vi "ActFollowRelativeTrajectory.vi"(7 "Orientation":T1, 9 "End Rotation":dbl, 10 "Trajectory":T2 {"States"."POSE"."ROTATION"."SIN" format="%13.4f"; "States"."POSE"."ROTATION"."COS" format="%13.4f"; "States"."POSE"."ROTATION"."VALUE" format="%13.4f"; "States"."POSE"."TRANSLATION"."Y" format="%14.3f"; "States"."POSE"."TRANSLATION"."X" format="%14.3f"; "TotalTImeSecs" format="%20.3f"}, 11 "FirstTime":bool) -> (0 "Done":bool, 1 "ASpeedDemand":dbl, 2 "YSpeedDemand":dbl, 3 "XSpeedDemand":dbl)   [LabVIEW 2020]
uses:
  <vilib>/Rock Robotics/WPI/ThirdParty/JAS_Junk/TrajLib/TypeDef/TRAJECTORY.ctl
  <vilib>/Rock Robotics/WPI/ThirdParty/JAS_Junk/TrajLib/TypeDef/TRAJ_STATE.ctl
  <vilib>/Rock Robotics/WPI/ThirdParty/JAS_Junk/TrajLib/TypeDef/POSE2D.ctl
  <vilib>/Rock Robotics/WPI/ThirdParty/JAS_Junk/TrajLib/TypeDef/TRANSLATION2D.ctl
  <vilib>/Rock Robotics/WPI/ThirdParty/JAS_Junk/TrajLib/TypeDef/ROTATION2D.ctl
  <vilib>/Rock Robotics/WPI/ThirdParty/JAS_Junk/TrajLib/Conv_Deg_Radians.vi
  <vilib>/Rock Robotics/WPI/ThirdParty/JAS_Junk/TrajLib/Rotation2d_CreateAngle.vi
  <vilib>/Rock Robotics/WPI/ThirdParty/JAS_Junk/TrajLib/Trajectory_Library.lvlib
  Autonomous/TrajectoryOrientation.ctl
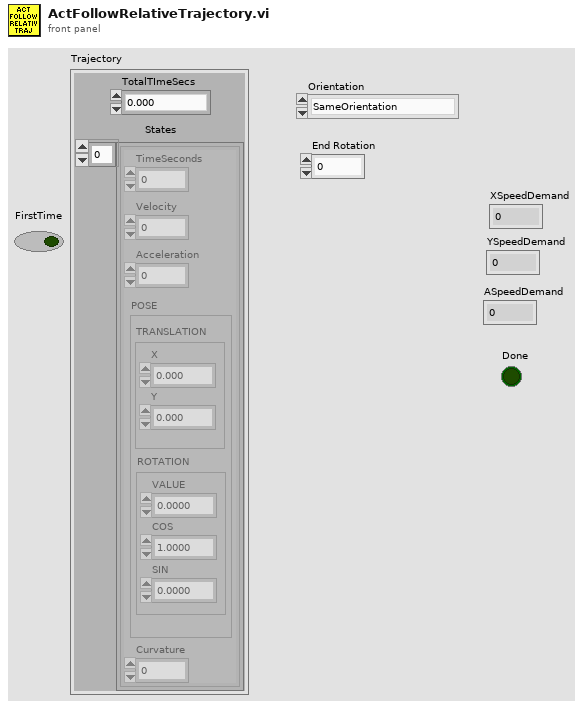
[diagram p1: front panel]
types:
  T1 = typedef "TrajectoryOrientation.ctl" = enum16{"SameOrientation", "RotateToEndOrientation"}
  T2 = typedef "Trajectory_Library.lvlib/TRAJECTORY.ctl" = cluster{"TotalTImeSecs":dbl, "States":T3[]}
  T3 = typedef "Trajectory_Library.lvlib/TRAJ_STATE.ctl" = cluster{"TimeSeconds":dbl, "Velocity":dbl, "Acceleration":dbl, "POSE":T4, "Curvature":dbl}
  T4 = typedef "Trajectory_Library.lvlib/POSE2D.ctl" = cluster{"TRANSLATION":T5, "ROTATION":T6}
  T5 = typedef "Trajectory_Library.lvlib/TRANSLATION2D.ctl" = cluster{"X":dbl, "Y":dbl}
  T6 = typedef "Trajectory_Library.lvlib/ROTATION2D.ctl" = cluster{"VALUE":dbl, "COS":dbl, "SIN":dbl}
  T7 = typedef "Trajectory_Library.lvlib/SWERVE_DRIVE_ODOMETRY.ctl" = cluster{"POSE":T4, "GyroOffset":T6, "PreviousAngle":T6, "PrevModulePositions":T8[], "NumModules":i32}
  T8 = typedef "Trajectory_Library.lvlib/SWERVE_DRIVE_MODULE_POSITION.ctl" = cluster{"Distance":dbl, "Angle":T6, "P":bool}
  T9 = typedef "Trajectory_Library.lvlib/SWERVE_DRIVE_KINEMATICS.ctl" = cluster{"NumModules":i32, "InverseKinematics":T10, "ForwardKinematics":T10, "Modules":T5[], "PrevCoR":T5, "SavedModuleStates":T11[]}
  T10 = typedef "NI_Matrix.lvlib/RealMatrix.ctl" = dbl[][]
  T11 = typedef "Trajectory_Library.lvlib/SWERVE_DRIVE_MODULE_STATE.ctl" = cluster{"Speed":dbl, "Angle":T6}
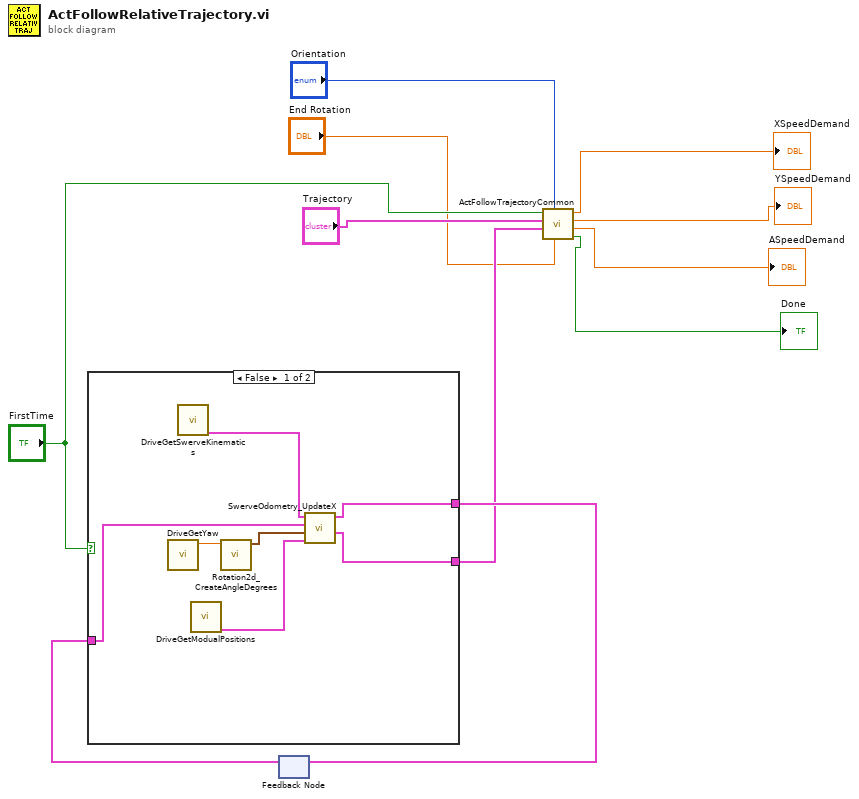
[diagram p0: block diagram]
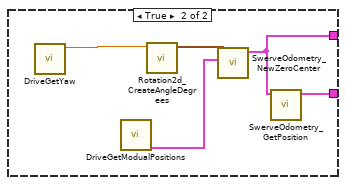
[diagram p2: hidden frame]
diagram:
  n1 = feedback #1() -> (w4:T7)  [unwired: 1 in]
  n2 = case shown="False" "FirstTime" {
    tunnel: [w13 w19] -> w5
    tunnel: w4 -> [w14 _]
    tunnel: [w12 w20] -> w3
    frame False {
      n3 = call "DriveGetYaw.vi"() -> ("Yaw"=w17:dbl)  [unwired: 11 in]
      n4 = call "DriveGetSwerveKinematics.vi"() -> ("SWERVE_DRIVE_KINEMATICS"=w15:T9)  [unwired: 11 in]
      n5 = call "DriveGetModualPositions.vi"() -> ("Swerve_Drive_Modual_Positions"=w18:T8[])  [unwired: 11 in]
      n6 = call <vilib>:"Rotation2d_CreateAngleDegrees.vi"("Angle_Degrees"=w17) -> ("ROTATION"=w16:T6)  [unwired: 10 in]
      n7 = call <vilib>:"SwerveOdometry_UpdateX.vi"("module Positions"=w18, "gyroAngle"=w16, "in SWERVE_DRIVE_ODOMETRY"=w14, "SWERVE_DRIVE_KINEMATICS"=w15) -> ("robot POSE"=w12:T4, "out SWERVE_DRIVE_ODOMETRY"=w13:T7)  [unwired: 5 in, 1 out]
    }
    frame True {
      n8 = call "DriveGetYaw.vi"() -> ("Yaw"=w23:dbl)  [unwired: 11 in]
      n9 = call "DriveGetModualPositions.vi"() -> ("Swerve_Drive_Modual_Positions"=w21:T8[])  [unwired: 11 in]
      n10 = call <vilib>:"Rotation2d_CreateAngleDegrees.vi"("Angle_Degrees"=w23) -> ("ROTATION"=w22:T6)  [unwired: 10 in]
      n11 = call <vilib>:"SwerveOdometry_NewZeroCenter.vi"("Module Positions"=w21, "gyroAngle"=w22) -> ("SWERVE_DRIVE_ODOMETRY"=w19:T7)  [unwired: 9 in]
      n12 = call <vilib>:"SwerveOdometry_GetPosition.vi"("in SWERVE_DRIVE_ODOMETRY"=w19) -> ("Pose"=w20:T4)  [unwired: 10 in]
    }
  }
  n13 = feedback-in #1(w5) -> ()
  n14 = call "ActFollowTrajectoryCommon.vi"("End Orientation"="End Rotation", "Orientation"="Orientation", "currentPose"=w3, "Trajectory"="Trajectory", "FirstTime"="FirstTime") -> ("Done"=→"Done":bool, "vAngularDemand"=→"ASpeedDemand":dbl, "vYSpeedDemand"=→"YSpeedDemand":dbl, "vXSpeedDemand"=→"XSpeedDemand":dbl)  [unwired: 3 in]
